vi "Conclude Call.vi"(8 "error in":errorcluster, 11 "ASE Handle":refnum<class "ase.lvclass">) -> (0 "error out":errorcluster, 1 "Exit Code":i32, 3 "Event References":T1)   [LabVIEW 2020, in "serenial.io-ase.lvlib" / "ase.lvclass"]
doc: "<B>Conclude the Asynchronous System Exec call.</B>\n\nThis VI waits for the call to finish and then deallocates internal resources.\n\n<B>This VI will still operate when there is an error at the error-in terminal.</B>\n\nThis VI generates the following errors:\n-5691000: Internal Library Error. Check Error Message for more details.\n1556: Invalid Handle Supplied"
uses:
  ase.lvclass
  Event References.ctl
  Standard Output.ctl
  Standard Error.ctl
  Did Exit.ctl
  ase.lvclass/ase.ctl
  Error Internal Library Implementation Error.vi
  <vilib>/Utility/error.llb/Error Cluster From Error Code.vi
  serenial.io-ase.32.dll
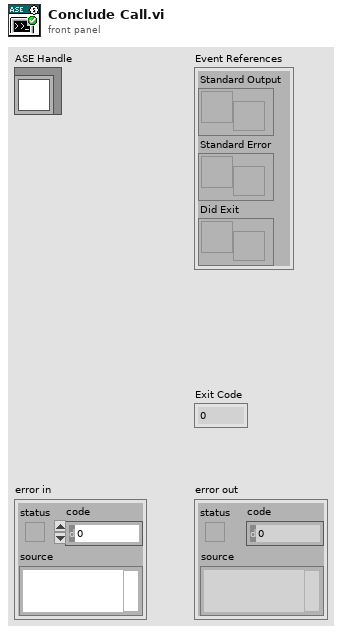
[diagram p1: front panel]
types:
  T1 = typedef "serenial.io-ase.lvlib/ase.lvclass/Event References.ctl" = cluster{"Standard Output":refnum<user-event>, "Standard Error":refnum<user-event>, "Did Exit":refnum<user-event>}
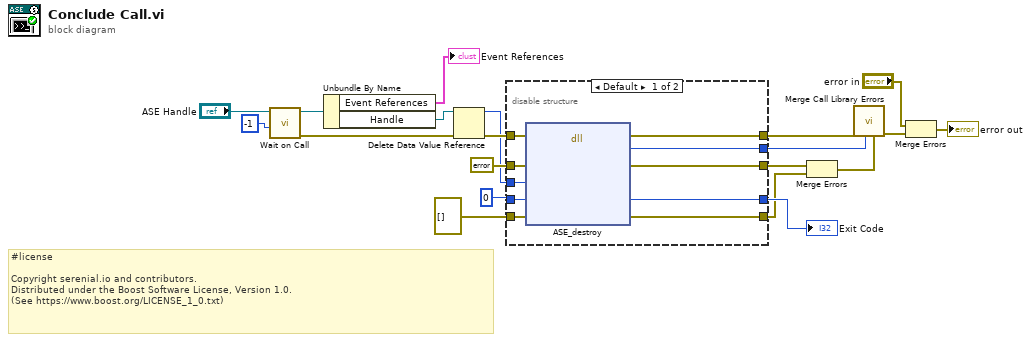
[diagram p0: block diagram]
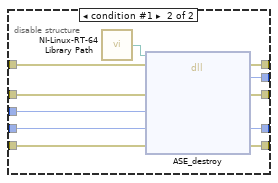
[diagram p2: hidden frame]
diagram:
  # "#license\n\nCopyright serenial.io and contributors.\nDistributed under the Boost Software License, Version 1.0.\n(See https://www.boost.org/LICENSE_1_0.txt)"
  n1 = call "Wait on Call.vi"("Timeout (ms)"=-1, "ASE Handle"="ASE Handle") -> ("error out"=w13:errorcluster, "ASE Handle Duplicate"=w14:refnum<class "ase.lvclass">)  [unwired: 7 in, 1 out]
  n2 = Unbundle By Name(w14) -> ("Event References"=→"Event References":T1, "Handle"=w11:refnum<data-value>)
  n3 = Delete Data Value Reference(data value reference=w11, error in=w13) -> (data value=w8:u64, error out=w10:errorcluster)
  n4 = disable-structure "Conditional Disable Structure" shown="Default" {
    disable-tunnel: w10 -> [w30 w40]
    disable-tunnel: errorcluster {"status"=FALSE, "code"=0, "source"=""} ("error") -> [w29 w34]
    disable-tunnel: w8 -> [w28 w35]
    disable-tunnel: 0 ("Exit Code") -> [w27 w36]
    disable-tunnel: errorcluster[] [] -> [w26 w37]
    disable-tunnel: [w25 w39] -> w5
    disable-tunnel: [w24 w38] -> w4
    disable-tunnel: [w23 w32] -> w3
    disable-tunnel: [w22 w33] -> w2
    disable-tunnel: [w21 w31] -> w1
    frame condition #0 (active) {
      n5 = dll-call lib="C:/serenial/libraries/Asynchronous-System-Executive/LabVIEW/serenial.io-ase/ase/serenial.io-ase.*.*" fn="ASE_destroy"(error in=w30, "Error Out"=w29, "ASE interface"=w28, "Exit Code"=w27, "Handler Errors"=w26) -> (error out=w25:errorcluster, "Error Code"=w24:i32, "Error Out"=w23:errorcluster, "Exit Code"=w22:i32, "Handler Errors"=w21:errorcluster[])  [unwired: 3 in, 1 out]
    }
    frame condition #1 {
      n6 = call "NI-Linux-RT-64 Library Path.vi"() -> ("Path"=w41:path)
      n7 = dll-call lib="?" fn="ASE_destroy"(path in=w41, error in=w40, "Error Out"=w34, "ASE interface"=w35, "Exit Code"=w36, "Handler Errors"=w37) -> (error out=w39:errorcluster, "Error Code"=w38:i32, "Error Out"=w32:errorcluster, "Exit Code"=w33:i32, "Handler Errors"=w31:errorcluster[])  [unwired: 2 in, 1 out]
    }
  }
  "Exit Code" <- w2
  n8 = Merge Errors(w3, w1) -> (w16:errorcluster)
  n9 = call "Merge Call Library Errors.vi"("Library Call Returned Error"=w16, "Error Code"=w4, "error in"=w5) -> ("error IO"=w18:errorcluster)  [unwired: 8 in]
  n10 = Merge Errors("error in", w18) -> (→"error out":errorcluster)
